vi "Scope Daemon.vi"(0 "Sciscan core Ref":path=path "C:/Users/Laa12/Desktop/SciScan_140404/GFG/GFG_core.ref", 1 "Buttons":T5, 2 "Indicators":T2, 3 "Visualization Parameters":T6, 5 "Current Frame":T1, 7 "Frame Time Stamp":refnum<vi>, 11 "error in (no error)":errorcluster, 12 "Transformation Matrix":refnum<vi>, 13 "FOV controls":T4, 14 "Parameters for Legal Movements":T3) -> (4 "Current Frame Out":T1, 15 "error out":errorcluster)   [LabVIEW 2012, in "Sciscan Scope Daemon.lvlib"]
uses:
  Sciscan Scope Daemon.lvlib
  <vilib>/Analysis/Matrix/Datatypes/RealMatrix.ctl
  <vilib>/vision/Image Controls.llb/IMAQ Image.ctl
  <vilib>/Analysis/Matrix/NI_Matrix.lvlib
panel:
  out "Exit":bool
  out "Image Out":T1
  out "FOVs":dbl[][](array[numeric])
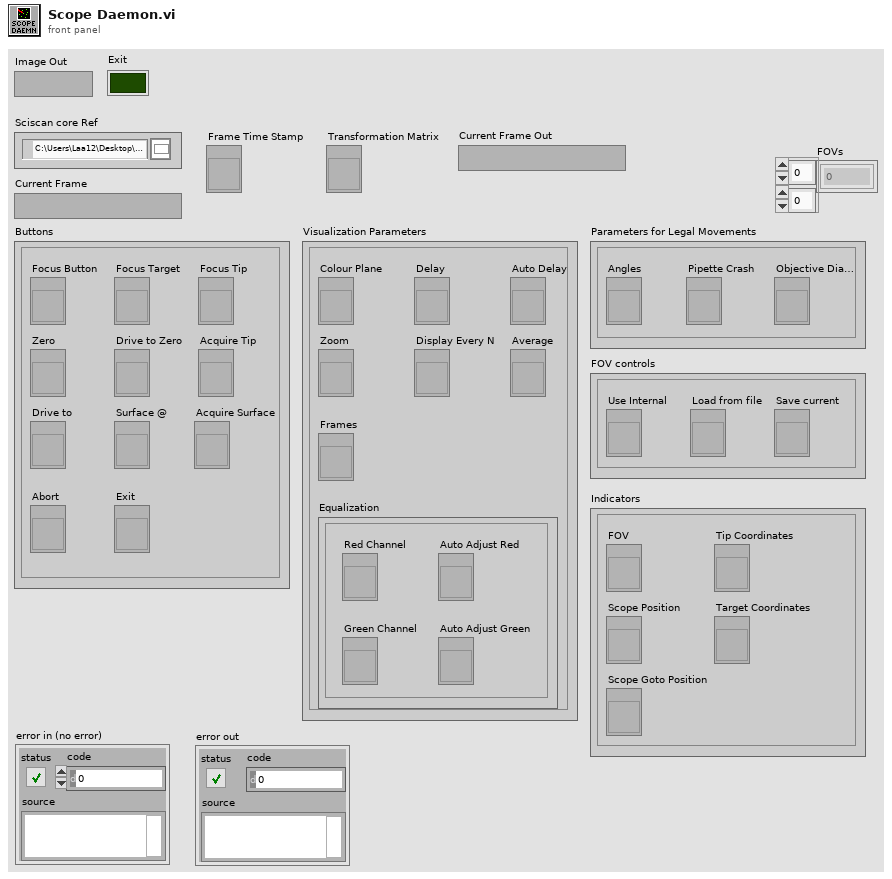
[diagram p1: front panel]
types:
  T1 = typedef "IMAQ Image.ctl" = refnum<image>
  T2 = cluster{"Tip Coordinates":refnum<vi>, "Target Coordinates":refnum<vi>, "Scope Position":refnum<vi>, "FOV":refnum<vi>, "Scope Goto Position":refnum<vi>}
  T3 = cluster{"Angles":refnum<vi>, "Objective Diameter":refnum<vi>, "Pipette Crash":refnum<vi>}
  T4 = cluster{"Use Internal":refnum<vi>, "Load from file":refnum<vi>, "Save current":refnum<vi>}
  T5 = cluster{"Focus Tip":refnum<vi>, "Focus Target":refnum<vi>, "Drive to Zero":refnum<vi>, "Zero":refnum<vi>, "Acquire Tip":refnum<vi>, "Focus Button":refnum<vi>, "Exit":refnum<vi>, "Abort":refnum<vi>, "Drive to":refnum<vi>, "Surface @":refnum<vi>, "Acquire Surface":refnum<vi>}
  T6 = cluster{"Display Every N":refnum<vi>, "Average":refnum<vi>, "Frames":refnum<vi>, "Colour Plane":refnum<vi>, "Zoom":refnum<vi>, "Delay":refnum<vi>, "Equalization":cluster{"Green Channel":refnum<vi>, "Auto Adjust Green":refnum<vi>, "Red Channel":refnum<vi>, "Auto Adjust Red":refnum<vi>}, "Auto Delay":refnum<vi>}
  T7 = cluster{"X [um]":dbl, "Y [um]":dbl, "Z [um]":dbl}
  T8 = typedef "NI_Matrix.lvlib/RealMatrix.ctl" = dbl[][]
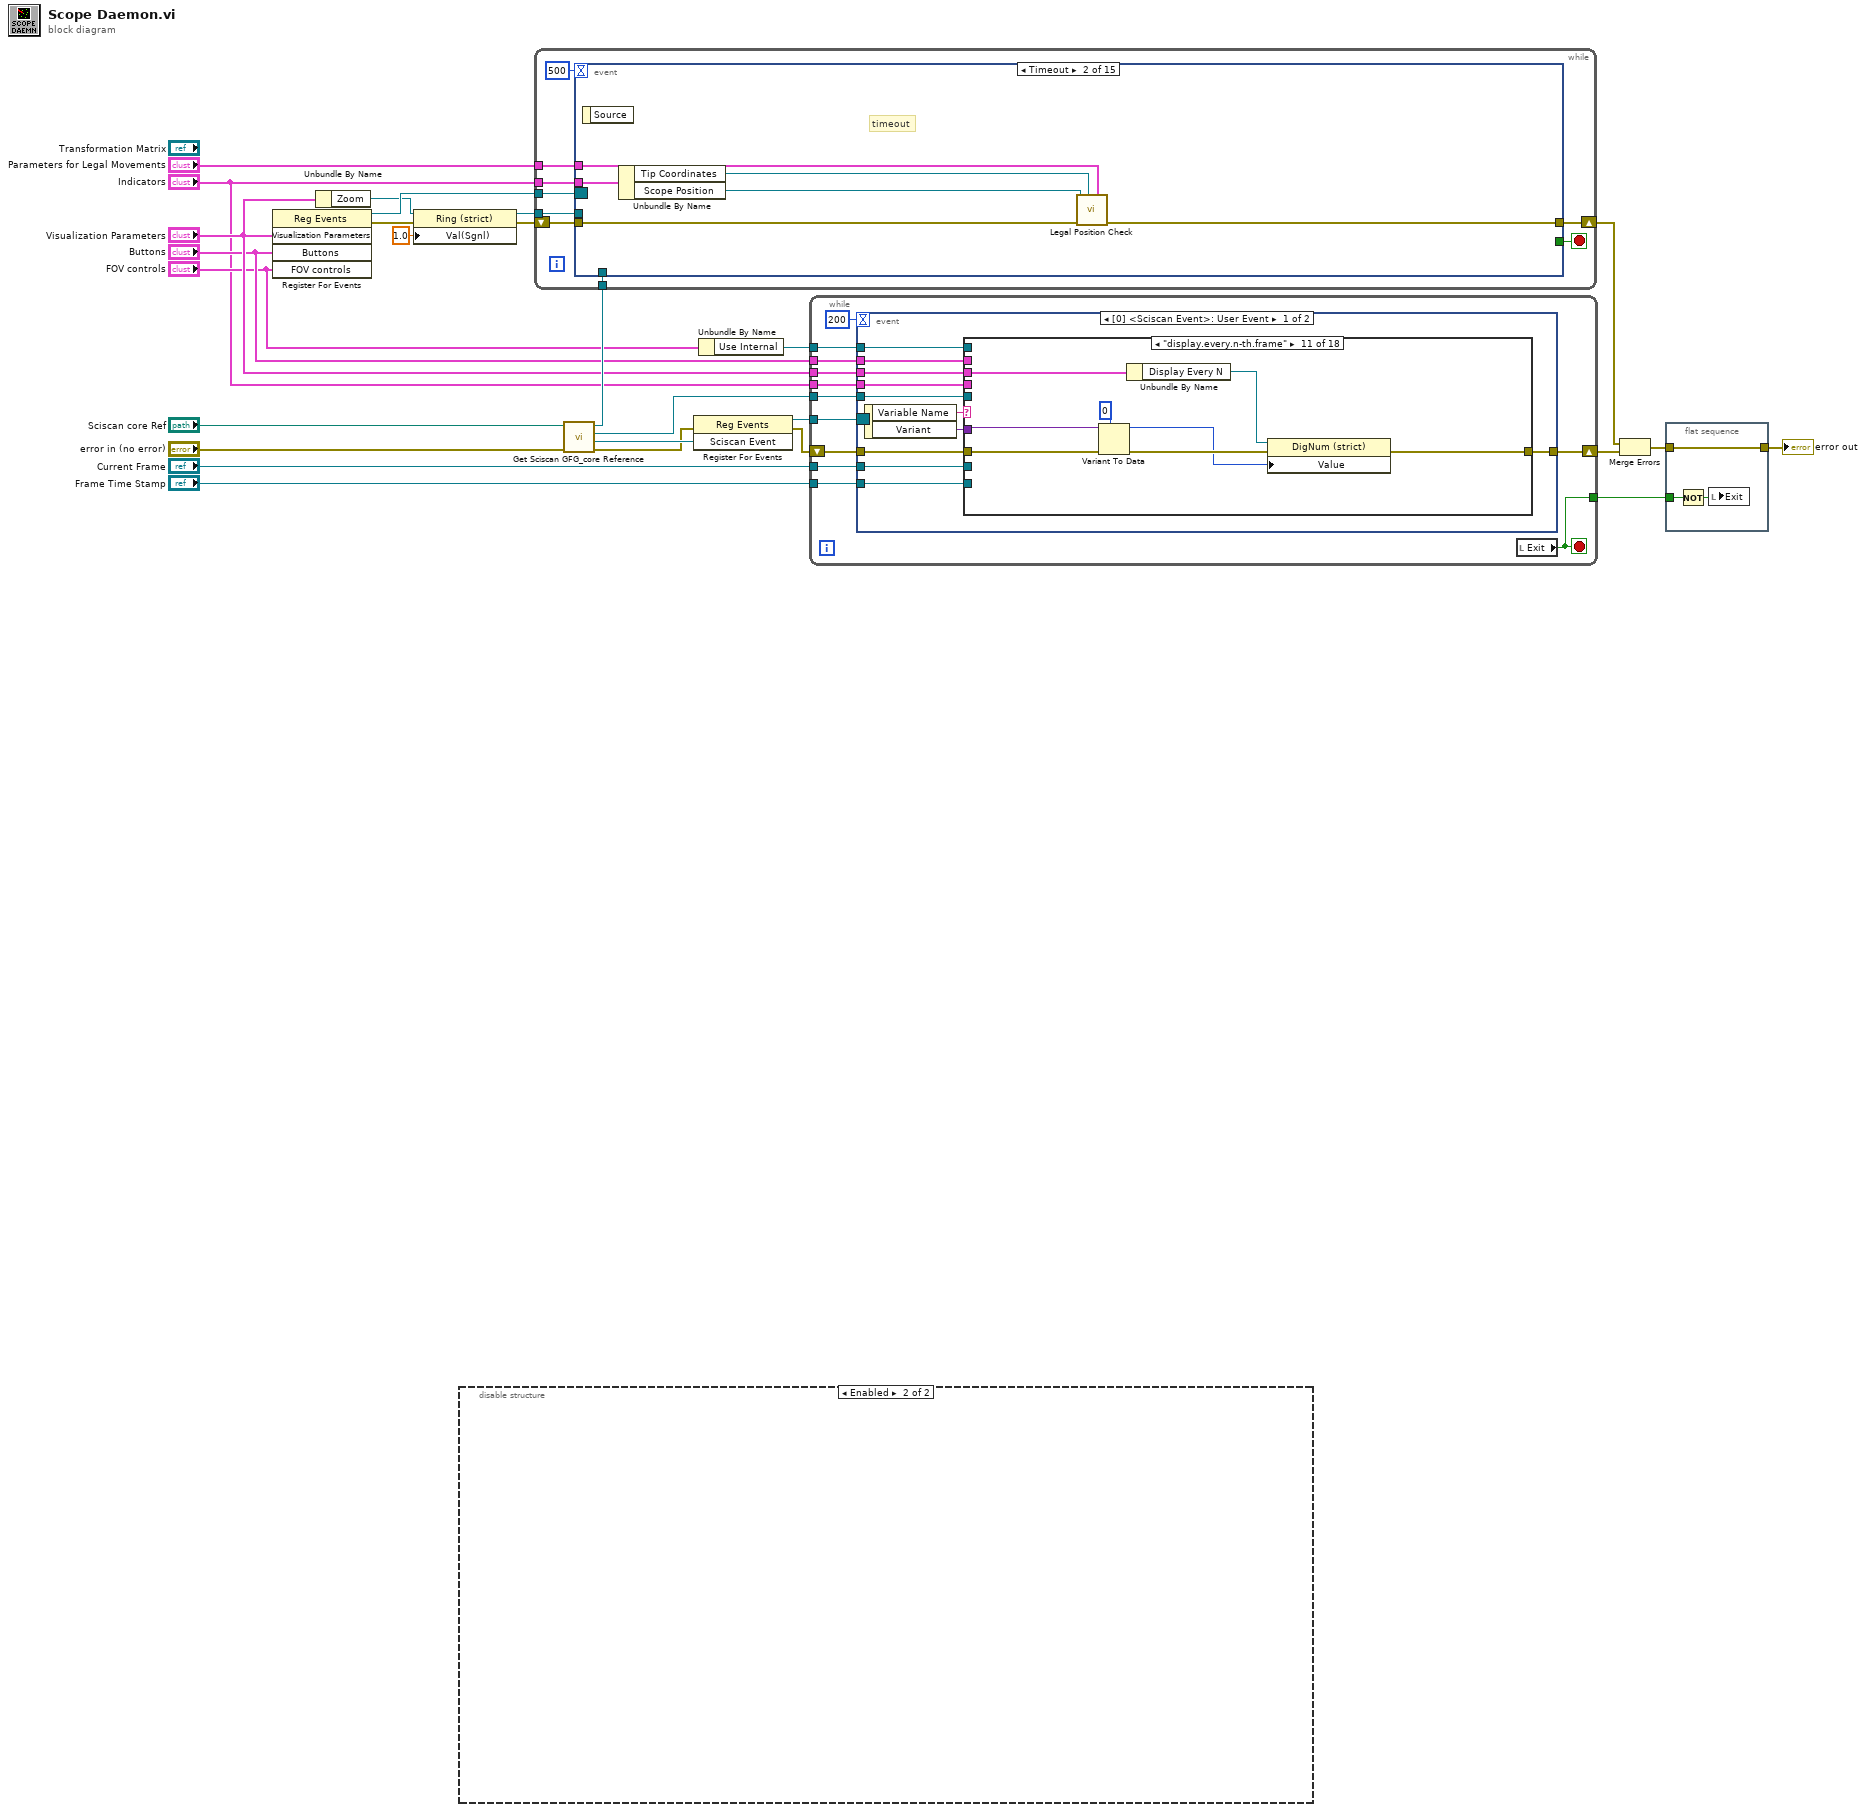
[diagram p0: block diagram]
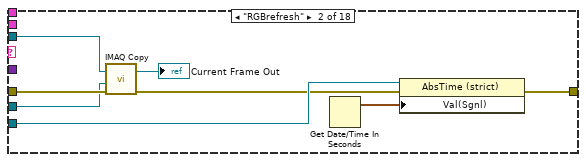
[diagram p3: hidden frame]
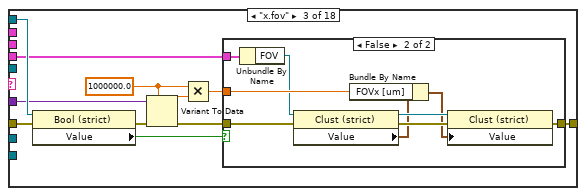
[diagram p4: hidden frame]
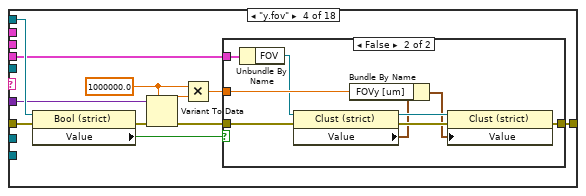
[diagram p6: hidden frame]
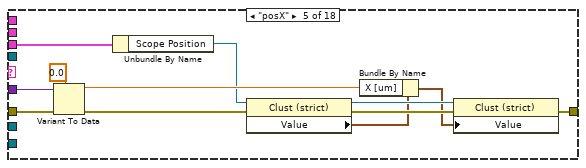
[diagram p8: hidden frame]
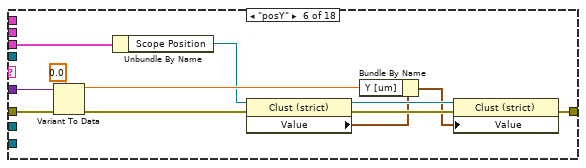
[diagram p9: hidden frame]
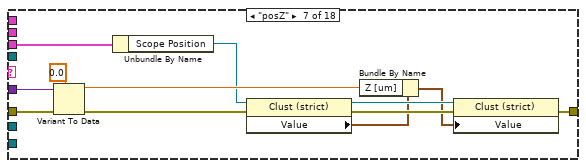
[diagram p10: hidden frame]
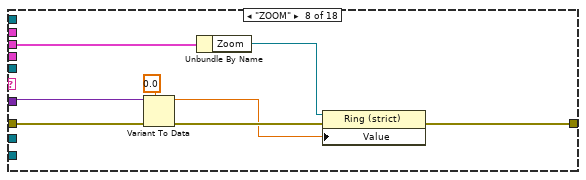
[diagram p11: hidden frame]
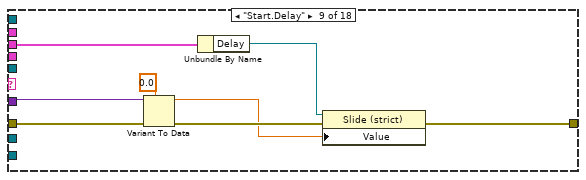
[diagram p12: hidden frame]
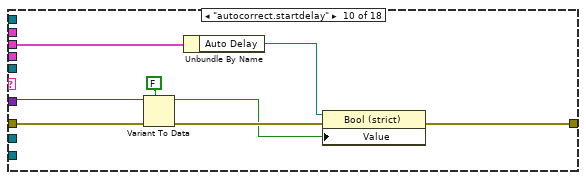
[diagram p13: hidden frame]
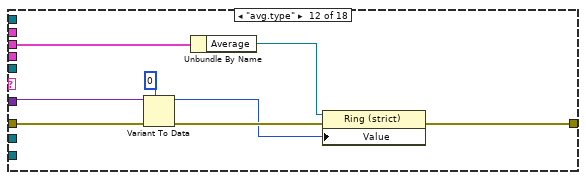
[diagram p14: hidden frame]
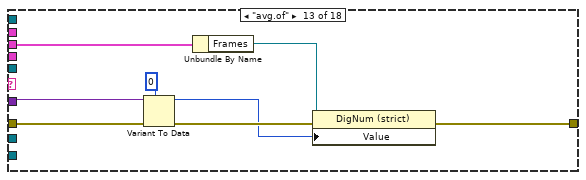
[diagram p15: hidden frame]
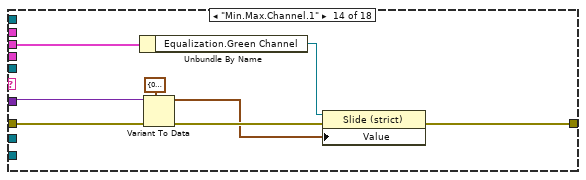
[diagram p16: hidden frame]
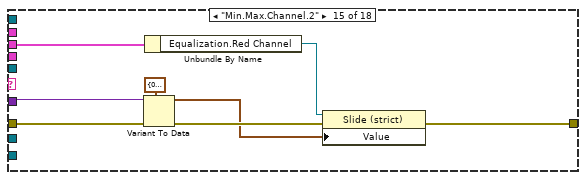
[diagram p17: hidden frame]
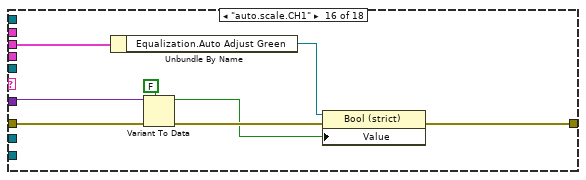
[diagram p18: hidden frame]
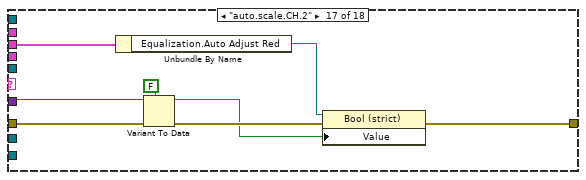
[diagram p19: hidden frame]
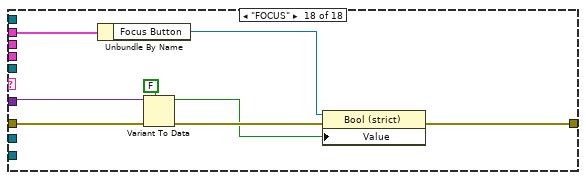
[diagram p20: hidden frame]
diagram:
  n1 = register-events("Visualization Parameters", "Buttons", "FOV controls") -> (reference out=w27:refnum<event-registration>, error out=w24:errorcluster)  [unwired: 2 in]
  n2 = Unbundle By Name("Visualization Parameters") -> ("Zoom"=w23:refnum<vi>)
  n3 = property class="Ring (strict)"(reference=w23, error in=w24, "Val(Sgnl)"=1.0 ("Value (Signaling)")) -> (reference out=w25:refnum<vi>, error out=w19:errorcluster)
  n4 = disable-structure shown="Enabled" {
    frame Disabled {
      n5 = List Folder(path=path "C:/Users/LAA12/Desktop/imagesRGB" ("Images Folder")) -> (path out=w37:path, filenames=w33:string[], error out=w30:errorcluster)  [unwired: 1 in, 3 out]
      n6 = call "IMAQ Create"("Image Name"="Current Image", "error in (no error)"=w30) -> ("New Image"=w40:T1, "error out"=w29:errorcluster)  [unwired: 2 in, 1 out]
      n7 = Delete From Array(array=w33, index=0) -> (array with subset deleted=w35:string[])  [unwired: 1 in, 1 out]
      n8 = Array Size(array=w35) -> (size(s)=w36:i32)
      n9 = Decrement(x=w36) -> (x-1=w32:i32)
      n10 = while {
        tunnel: w40 -> [w55]
        tunnel: w32 -> [w45]
        shift-right: [w50] -> _
        shift-left: u32 0 -> [w47]
        shift-right: [w43] -> w34
        shift-left: w29 -> [w58]
        tunnel: w37 -> [w57]
        tunnel: w35 -> [w56]
        tunnel: [w44] -> w28
        stop <- FALSE stop-if-true
        n11 = Index Array(array=w56, index=w47) -> (element=w54:string)
        n12 = Increment(x=w47) -> (x+1=w46:u32)
        n13 = Build Path(base path=w57, name or relative path=w54) -> (appended path=w53:path)
        n14 = call "IMAQ ReadFile"("File Path"=w53, "error in (no error)"=w58, "Image"=w55) -> ("error out"=w43:errorcluster, "Image Out"=w44:T1)  [unwired: 2 in, 5 out]
        "Image Out" <- w44
        n15 = Less?(x=w46, y=w45) -> (x < y?=w52:bool)
        n16 = Wait (ms)(milliseconds to wait=u32 500) -> ()  [unwired: 1 out]
        n17 = Select(t=w46, s=w52, f=u32 0) -> (s? t:f=w50:u32)
      }
      n18 = call "IMAQ Dispose"("Image"=w28, "error in (no error)"=w34) -> ("error out"=w41:errorcluster)  [unwired: 1 in, 3 out]
      n19 = call <vilib>:"Simple Error Handler.vi"("error in (no error)"=w41) -> ()  [unwired: 1 in, 8 out]
    }
    frame Enabled {
    }
  }
  n20 = call "Get Sciscan GFG_core Reference.vi"("error in"="error in (no error)", "file path"="Sciscan core Ref") -> ("error out"=w10:errorcluster, "Sciscan Event"=w11:refnum<user-event>, "RGB overlay"=w14:T1, "GFG reference"=w17:refnum<vi>)  [unwired: 6 in]
  n21 = while {
    tunnel: w27 -> [w67]
    shift-right: [w66] -> w4
    shift-left: w19 -> [w65]
    tunnel: w25 -> [w63]
    tunnel: w17 -> [w59]
    tunnel: "Parameters for Legal Movements" -> [w61]
    tunnel: "Indicators" -> [w60]
    stop <- w64 stop-if-true
    n22 = event shown="[1] Timeout" {
      selector: w67 -> [_ _ _ _ _ _ _ _ _ _ _ _ _ _ _]
      dyn-events: _ -> [_ _ _ _ _ _ _ _ _ _ _ _ _ _ _]
      timeout: 500 -> [_ _ _ _ _ _ _ _ _ _ _ _ _ _ _]
      tunnel: [w74 w94 w108 w117 w137 w143 w198 w214 w231 w242 w246 w250 w252 w267 w271] -> w66
      tunnel: w65 -> [w71 w99 w103 w116 w134 w146 w199 w213 w239 w243 w245 w251 w255 w259 w271]
      tunnel: [_ _ _ _ _ _ _ _ _ _ _ _ _ _ TRUE] -> w64
      tunnel: w63 -> [_ _ _ _ _ w144 _ _ _ _ _ _ _ _ _]
      tunnel: w61 -> [_ w98 _ _ _ _ _ _ _ _ _ _ _ _ _]
      tunnel: w60 -> [_ w97 _ _ _ _ _ _ _ _ _ _ _ w262 _]
      tunnel: w59 -> [w73 _ w104 w115 w135 w145 _ w212 w229 w241 w247 w249 w254 _ _]
      event Value Change {
        # "dynamics"
        # "focus target\nfocus tip"
        n23 = event-data() -> ("CtlRef"=w75:refnum<vi>)  [unwired: 1 in]
        n24 = local read "Visualization Parameters"() -> (w70:T6)
        n25 = local read "Buttons"() -> (w77:T5)
        n26 = local read "Indicators"() -> (w79:T2)
        n27 = Unbundle By Name(w70) -> ("Zoom"=w69:refnum<vi>)
        n28 = Unbundle By Name(w77) -> ("Focus Target"=w78:refnum<vi>)
        n29 = Unbundle By Name(w79) -> ("Target Coordinates"=w82:refnum<vi>, "Tip Coordinates"=w83:refnum<vi>, "FOV"=w84:refnum<vi>)
        n30 = property class="Ring (strict)"(reference=w69, error in=w71) -> (error out=w72:errorcluster, "Value"=w68:dbl)  [unwired: 1 out]
        n31 = local read "Transformation Matrix"() -> (w76:refnum<vi>)
        n32 = property class="Clust (strict)"(reference=w84) -> (error out=w93:errorcluster, "Value"=w86:cluster{"FOVx [um]":dbl, "FOVy [um]":dbl})  [unwired: 1 in, 1 out]
        n33 = Equal?(x=w78, y=w75) -> (x = y?=w92:bool)
        n34 = Select(t=w82, s=w92, f=w83) -> (s? t:f=w90:refnum<vi>)
        n35 = property class="Clust (strict)"(reference=w90, error in=w93) -> (error out=w89:errorcluster, "Value"=w85:T7)  [unwired: 1 out]
        n36 = property class="Arr (strict)"(reference=w76, error in=w72) -> (error out=w81:errorcluster, "Value"=w80:T8)  [unwired: 1 out]
        n37 = call "Focus Point.vi"("Zoom Factor"=w68, "Transformation Matrix"=w80, "error in"=w81, "FOV"=w86, "Target Coordinates"=w85, "GFG Refnum"=w73) -> ("error out"=w91:errorcluster)  [unwired: 4 in, 1 out]
        n38 = property class="Bool (strict)"(reference=w75, error in=w89, "Value"=FALSE) -> (error out=w87:errorcluster)  [unwired: 1 out]
        n39 = Merge Errors(w87, w91) -> (w74:errorcluster)
      }
      event Timeout {
        # "timeout"
        n40 = event-data() -> ()  [unwired: 1 in, 1 out]
        n41 = Unbundle By Name(w97) -> ("Tip Coordinates"=w96:refnum<vi>, "Scope Position"=w95:refnum<vi>)
        n42 = call "Legal Position Check.vi"("Parameters for Legal Movements"=w98, "error in (no error)"=w99, "Scope Position"=w95, "Tip Coordinates"=w96) -> ("error out"=w94:errorcluster)  [unwired: 6 in, 1 out]
      }
      event Value Change {
        # "drive to position"
        n43 = event-data() -> ()  [unwired: 1 in, 3 out]
        n44 = call "Set Sciscan Dynamics.vi"("error in"=w103, "Fast"=FALSE, "GFG Refnum"=w104) -> ("error out"=w102:errorcluster, "GFG Refnum Out"=w101:refnum<vi>)  [unwired: 7 in]
        n45 = local read "Buttons"() -> (w107:T5)
        n46 = local read "Indicators"() -> (w113:T2)
        n47 = Unbundle By Name(w107) -> ("Drive to"=w106:refnum<vi>)
        n48 = Unbundle By Name(w113) -> ("Scope Goto Position"=w112:refnum<vi>)
        n49 = property on="Property Node" class="Clust (strict)"(reference=w112, error in=w102) -> (error out=w111:errorcluster, "Value"=w110:T7)  [unwired: 1 out]
        n50 = call "Move Sciscan Scope.vi"("Type"=enum16{"Relative", "Absolute"}."Absolute", "error in"=w111, "Displacement [um]"=w110, "GFG Refnum"=w101) -> ("error out"=w109:errorcluster)  [unwired: 6 in, 1 out]
        n51 = property on="Property Node" class="Bool (strict)"(reference=w106, error in=w109, "Value"=FALSE) -> (error out=w108:errorcluster)  [unwired: 1 out]
      }
      event Value Change {
        # "zero"
        n52 = event-data() -> ("CtlRef"=w118:refnum<vi>)  [unwired: 1 in]
        n53 = flat-sequence {
          tunnel: w116 -> [w125]
          tunnel: w115 -> [w126]
          tunnel: [w126] -> w123
          tunnel: [w125] -> w122
          tunnel: [w127] -> w121
          tunnel: w123 -> [w129]
          tunnel: w122 -> [w128]
          tunnel: [w131] -> w120
          tunnel: w121 -> [w131]
          frame #0 {
            n54 = Wait (ms)(milliseconds to wait=u32 1000) -> ()  [unwired: 1 out]
          }
          frame #1 {
            n55 = call "Zero.vi"("error in"=w128, "GFG Refnum"=w129) -> ("error out"=w127:errorcluster)  [unwired: 8 in, 1 out]
          }
          frame #2 {
            n56 = Wait (ms)(milliseconds to wait=u32 2000) -> ()  [unwired: 1 out]
          }
        }
        n57 = property on="Property Node" class="Bool (strict)"(reference=w118, error in=w120, "Value"=FALSE) -> (error out=w117:errorcluster)  [unwired: 1 out]
      }
      event Value Change {
        # "dynamics"
        # "drive to zero"
        n58 = event-data() -> ("CtlRef"=w138:refnum<vi>)  [unwired: 1 in]
        n59 = call "Set Sciscan Dynamics.vi"("error in"=w134, "Fast"=FALSE, "GFG Refnum"=w135) -> ("error out"=w133:errorcluster, "GFG Refnum Out"=w132:refnum<vi>)  [unwired: 7 in]
        n60 = call "Move Sciscan Scope.vi"("Type"=enum16{"Relative", "Absolute"}."Absolute", "error in"=w133, "Displacement [um]"=T7 {"X [um]"=0.0, "Y [um]"=0.0, "Z [um]"=0.0}, "GFG Refnum"=w132) -> ("error out"=w140:errorcluster)  [unwired: 6 in, 1 out]
        n61 = property on="Property Node" class="Bool (strict)"(reference=w138, error in=w140, "Value"=FALSE) -> (error out=w137:errorcluster)  [unwired: 1 out]
      }
      event Value Change {
        # "zoom\nuse internal"
        n62 = event-data() -> ()  [unwired: 1 in, 1 out]
        n63 = local read "FOV controls"() -> (w151:T4)
        n64 = Unbundle By Name(w151) -> ("Use Internal"=w150:refnum<vi>)
        n65 = property class="Ring (strict)"(reference=w144, error in=w146) -> (reference out=w152:refnum<vi>, error out=w160:errorcluster, "Value"=w159:dbl)
        n66 = property class="Bool (strict)"(reference=w150) -> (error out=w147:errorcluster, "Value"=w153:bool)  [unwired: 1 in, 1 out]
        n67 = call "Set Sciscan Scope Zoom.vi"("error in"=w160, "Zoom"=w159, "GFG Refnum"=w145) -> ("error out"=w156:errorcluster, "GFG Refnum Out"=w155:refnum<vi>)  [unwired: 7 in]
        n68 = case shown="False" w153 {
          tunnel: w155 -> [w166 _]
          tunnel: [w165 w175] -> w149
          tunnel: w156 -> [w164 w178]
          tunnel: [w161 w186] -> w158
          tunnel: w152 -> [_ w185]
          frame False {
            n69 = flat-sequence {
              tunnel: w164 -> [w168]
              tunnel: w166 -> [w169]
              tunnel: [w169] -> w163
              tunnel: [w168] -> w162
              tunnel: [w172] -> w165
              tunnel: [w170] -> w161
              tunnel: w163 -> [w173]
              tunnel: w162 -> [w171]
              frame #0 {
                n70 = Wait (ms)(milliseconds to wait=u32 2000) -> ()  [unwired: 1 out]
              }
              frame #1 {
                n71 = call "Get Sciscan FOV.vi"("error in"=w171, "GFG Refnum"=w173) -> ("error out"=w172:errorcluster, "FOV"=w170:cluster{"Width [um]":dbl, "Height [um]":dbl})  [unwired: 7 in, 1 out]
              }
            }
          }
          frame True {
            w183 = 0 ("index (row)")
            n72 = local read "FOVs"() -> (w174:dbl[][])
            n73 = Index Array(array=w174, index (row)=w183, index (col)=w183) -> (element=w182:dbl)
            n74 = Not A Number/Path/Refnum?(number/path/refnum=w182) -> (NaN/Path/Refnum?=w181:bool)
            n75 = Less Or Equal To 0?(x=w182) -> (x <= 0?=w180:bool)
            n76 = Or(x=w181, y=w180) -> (x .or. y?=w179:bool)
            n77 = case shown="True" w179 {
              tunnel: [w193 w196] -> w177
              tunnel: w178 -> [w193 w195]
              tunnel: [w192 w194] -> w176
              tunnel: w174 -> [w192 _]
              frame False {
              }
              frame True {
                n78 = call "Load Zoom FOV table.vi"("error in"=w195, "Max Zoom"=8) -> ("error out"=w196:errorcluster, "FOVs"=w194:dbl[][])  [unwired: 8 in]
              }
            }
            "FOVs" <- w176
            n79 = property on="Property Node" class="Ring (strict)"(reference=w185, error in=w177) -> (error out=w175:errorcluster, "Value"=w191:dbl)  [unwired: 1 out]
            n80 = Decrement(x=w191) -> (x-1=w184:dbl)
            n81 = Index Array(array=w176, index (row) #1=w184, index (col) #1=1 ("disabled index (col)"), index (row) #2=w184, index (col) #2=2 ("disabled index (col)")) -> (element #1=w188:dbl, element #2=w187:dbl)
            n82 = Bundle("input 3"=w188, "input 3"=w187) -> (w186:cluster{"input 3":dbl, "input 3":dbl})  [unwired: 1 in]
          }
        }
        n83 = local read "Indicators"() -> (w154:T2)
        n84 = Unbundle By Name(w154) -> ("FOV"=w157:refnum<vi>)
        n85 = property on="Property Node" class="Clust (strict)"(reference=w157, error in=w149, "Value"=w158) -> (error out=w148:errorcluster)  [unwired: 1 out]
        n86 = Merge Errors(w147, w148) -> (w143:errorcluster)
      }
      event Value Change {
        # "load from file"
        n87 = event-data() -> ("CtlRef"=w200:refnum<vi>)  [unwired: 1 in]
        n88 = local read "Visualization Parameters"() -> (w201:T6)
        n89 = local read "Indicators"() -> (w210:T2)
        n90 = Unbundle By Name(w201) -> ("Zoom"=w207:refnum<vi>)
        n91 = Unbundle By Name(w210) -> ("FOV"=w209:refnum<vi>)
        n92 = property class="Clust (strict)"(reference=w209, error in=w199) -> (error out=w208:errorcluster, "Value"=w204:cluster{"FOVx [um]":dbl, "FOVy [um]":dbl})  [unwired: 1 out]
        n93 = property class="Ring (strict)"(reference=w207, error in=w208) -> (error out=w205:errorcluster, "Value"=w206:dbl)  [unwired: 1 out]
        n94 = call "Save Current Fov.vi"("Max Zoom"=8, "error in"=w205, "Current FOV"=w204, "Current Zoom"=w206) -> ("error out"=w203:errorcluster)  [unwired: 6 in, 1 out]
        n95 = property class="Bool (strict)"(reference=w200, error in=w203, "Value"=FALSE) -> (error out=w198:errorcluster)  [unwired: 1 out]
      }
      event Value Change {
        n96 = event-data() -> ()  [unwired: 1 in, 1 out]
        n97 = local read "Visualization Parameters"() -> (w228:T6)
        n98 = Unbundle By Name(w228) -> ("Equalization.Red Channel"=w225:refnum<vi>, "Equalization.Green Channel"=w226:refnum<vi>, "Equalization.Auto Adjust Green"=w221:refnum<vi>, "Equalization.Auto Adjust Red"=w220:refnum<vi>)
        n99 = property class="Slide (strict)"(reference=w226) -> (error out=w227:errorcluster, "Value"=w223:cluster{dbl, dbl})  [unwired: 1 in, 1 out]
        n100 = property class="Bool (strict)"(reference=w220) -> (error out=w222:errorcluster, "Value"=w218:bool)  [unwired: 1 in, 1 out]
        n101 = property class="Slide (strict)"(reference=w225, error in=w227) -> (error out=w216:errorcluster, "Value"=w224:cluster{dbl, dbl})  [unwired: 1 out]
        n102 = property class="Bool (strict)"(reference=w221, error in=w222) -> (error out=w217:errorcluster, "Value"=w219:bool)  [unwired: 1 out]
        n103 = call "Set Sciscan Scope Image Equalization.vi"("Red Channel"=w224, "Green Channel"=w223, "error in"=w213, "Auto Adjust Red"=w218, "Auto Adjust Green"=w219, "GFG Refnum"=w212) -> ("error out"=w215:errorcluster)  [unwired: 4 in, 1 out]
        n104 = Merge Errors(w216, w217, w215) -> (w214:errorcluster)
      }
      event Value Change {
        # "avg\nframes"
        n105 = event-data() -> ()  [unwired: 1 in, 1 out]
        n106 = local read "Visualization Parameters"() -> (w238:T6)
        n107 = Unbundle By Name(w238) -> ("Average"=w237:refnum<vi>, "Frames"=w236:refnum<vi>)
        n108 = property class="DigNum (strict)"(reference=w236) -> (error out=w235:errorcluster, "Value"=w233:i8)  [unwired: 1 in, 1 out]
        n109 = property class="Ring (strict)"(reference=w237, error in=w235) -> (error out=w230:errorcluster, "Value"=w234:u16)  [unwired: 1 out]
        n110 = call "Set Sciscan Scope Image Averaging.vi"("error in"=w239, "Frames"=w233, "Average"=w234, "GFG Refnum"=w229) -> ("error out"=w232:errorcluster)  [unwired: 6 in, 1 out]
        n111 = Merge Errors(w230, w232) -> (w231:errorcluster)
      }
      event Value Change {
        # "display every N"
        n112 = event-data() -> ("NewVal"=w240:i8)  [unwired: 1 in]
        n113 = call "Set Sciscan Scope Image Refresh.vi"("error in"=w243, "display every n-th frame"=w240, "GFG Refnum"=w241) -> ("error out"=w242:errorcluster)  [unwired: 7 in, 1 out]
      }
      event Value Change {
        # "Delay"
        n114 = event-data() -> ("NewVal"=w244:dbl)  [unwired: 1 in]
        n115 = call "Set Sciscan Scope Image Delay.vi"("error in"=w245, "Delay"=w244, "GFG Refnum"=w247) -> ("error out"=w246:errorcluster)  [unwired: 7 in, 1 out]
      }
      event Value Change {
        # "Delay"
        n116 = event-data() -> ("NewVal"=w248:bool)  [unwired: 1 in]
        n117 = call "Auto Sciscan Scope Image Delay.vi"("error in"=w251, "Auto Delay"=w248, "GFG Refnum"=w249) -> ("error out"=w250:errorcluster)  [unwired: 7 in, 1 out]
      }
      event Value Change {
        # "focus"
        n118 = event-data() -> ("NewVal"=w253:bool)  [unwired: 1 in]
        n119 = call "Set Sciscan Scope Focus.vi"("error in"=w255, "Focus Button"=w253, "GFG Refnum"=w254) -> ("error out"=w252:errorcluster)  [unwired: 7 in, 1 out]
      }
      event "Buttons.Acquire Surface": Value Change {
        n120 = event-data() -> ()  [unwired: 1 in, 1 out]
        n121 = local read "Buttons"() -> (w266:T5)
        n122 = Unbundle By Name(w266) -> ("Acquire Surface"=w265:refnum<vi>, "Surface @"=w261:refnum<vi>)
        n123 = Unbundle By Name(w262) -> ("Scope Position"=w258:refnum<vi>)
        n124 = property on="Property Node" class="Clust (strict)"(reference=w258, error in=w259) -> (error out=w260:errorcluster, "Value"=w257:T7)  [unwired: 1 out]
        n125 = Unbundle By Name(w257) -> ("Z [um]"=w256:dbl)
        n126 = property on="Property Node" class="DigNum (strict)"(reference=w261, error in=w260, "Value"=w256) -> (error out=w263:errorcluster)  [unwired: 1 out]
        n127 = property on="Property Node" class="Bool (strict)"(reference=w265, error in=w263, "Value"=FALSE) -> (error out=w267:errorcluster)  [unwired: 1 out]
      }
      event Value Change {
        # "exit"
        n128 = event-data() -> ()  [unwired: 1 in, 1 out]
        n129 = local write "FOVs"(dbl[][] [] ("Array")) -> ()
        "Exit" <- TRUE ("Exit")
      }
    }
  }
  n130 = register-events(error in=w10, w11) -> (reference out=w18:refnum<event-registration>, error out=w12:errorcluster)  [unwired: 1 in]
  n131 = Unbundle By Name("FOV controls") -> ("Use Internal"=w16:refnum<vi>)
  n132 = while {
    tunnel: w18 -> [w283]
    tunnel: w16 -> [w282]
    shift-right: [w280] -> w5
    shift-left: w12 -> [w281]
    tunnel: "Indicators" -> [w279]
    tunnel: "Visualization Parameters" -> [w278]
    tunnel: "Frame Time Stamp" -> [w277]
    tunnel: w14 -> [w276]
    tunnel: "Current Frame" -> [w275]
    tunnel: "Buttons" -> [w274]
    tunnel: [w273] -> w1
    stop <- w273 stop-if-true
    n133 = event shown="[0] <Sciscan Event>: User Event" {
      selector: w283 -> [_ _]
      dyn-events: _ -> [_ _]
      timeout: 200 -> [_ _]
      tunnel: w282 -> [w293 _]
      tunnel: w281 -> [w292 w470]
      tunnel: [w291 w470] -> w280
      tunnel: w279 -> [w290 _]
      tunnel: w278 -> [w289 _]
      tunnel: w277 -> [w287 _]
      tunnel: w276 -> [w286 _]
      tunnel: w275 -> [w285 _]
      tunnel: w274 -> [w284 _]
      event User Event {
        n134 = event-data() -> ("Variable Name"=w288:string, "Variant"=w294:variant)  [unwired: 1 in]
        n135 = case shown="\"display.every.n-th.frame\"" w288 {
          tunnel: w294 -> [_ _ w311 w332 w357 w369 w381 w388 w396 w404 w412 w420 w428 w436 w444 w452 w460 w468]
          tunnel: w293 -> [_ _ w313 w334 _ _ _ _ _ _ _ _ _ _ _ _ _ _]
          tunnel: w292 -> [w295 w301 w312 w333 w346 w358 w370 w389 w397 w405 w413 w421 w429 w437 w445 w453 w461 w469]
          tunnel: [w295 w302 w306 w327 w355 w367 w379 w386 w394 w402 w410 w418 w426 w434 w442 w450 w458 w466] -> w291
          tunnel: w290 -> [_ _ w304 w325 w354 w366 w378 _ _ _ _ _ _ _ _ _ _ _]
          tunnel: w289 -> [_ _ _ _ _ _ _ w385 w393 w401 w409 w417 w425 w433 w441 w449 w457 _]
          tunnel: w287 -> [_ w303 _ _ _ _ _ _ _ _ _ _ _ _ _ _ _ _]
          tunnel: w286 -> [_ w300 _ _ _ _ _ _ _ _ _ _ _ _ _ _ _ _]
          tunnel: w285 -> [_ w299 _ _ _ _ _ _ _ _ _ _ _ _ _ _ _ _]
          tunnel: w284 -> [_ _ _ _ _ _ _ _ _ _ _ _ _ _ _ _ _ w462]
          frame "False", Default {
          }
          frame "RGBrefresh" {
            n136 = call "IMAQ Copy"("error in (no error)"=w301, "Image Dst"=w299, "Image Src"=w300) -> ("error out"=w297:errorcluster, "Image Dst Out"=→"Current Frame Out":T1)  [unwired: 3 out]
            n137 = Get Date/Time In Seconds() -> (seconds since 1Jan1904=w298:timestamp)
            n138 = property on="Property Node" class="AbsTime (strict)"(reference=w303, error in=w297, "Val(Sgnl)"=w298) -> (error out=w302:errorcluster)  [unwired: 1 out]
          }
          frame "x.fov" {
            w308 = 1000000.0
            n139 = property class="Bool (strict)"(reference=w313, error in=w312) -> (error out=w310:errorcluster, "Value"=w314:bool)  [unwired: 1 out]
            n140 = Variant To Data(error in=w310, type=w308, Variant=w311) -> (data=w305:dbl, error out=w309:errorcluster)
            n141 = Multiply(x=w308, y=w305) -> (x*y=w307:dbl)
            n142 = case shown="False" w314 {
              tunnel: [w315 w324] -> w306
              tunnel: w309 -> [w315 w323]
              tunnel: w307 -> [_ w320]
              tunnel: w304 -> [_ w316]
              frame True {
              }
              frame False {
                n143 = Unbundle By Name(w316) -> ("FOV"=w317:refnum<vi>)
                n144 = property on="Property Node" class="Clust (strict)"(reference=w317, error in=w323) -> (reference out=w321:refnum<vi>, error out=w322:errorcluster, "Value"=w319:cluster{"FOVx [um]":dbl, "FOVy [um]":dbl})
                n145 = Bundle By Name(cluster=w319, "FOVx [um]"=w320) -> (w318:cluster{"FOVx [um]":dbl, "FOVy [um]":dbl})
                n146 = property on="Property Node" class="Clust (strict)"(reference=w321, error in=w322, "Value"=w318) -> (error out=w324:errorcluster)  [unwired: 1 out]
              }
            }
          }
          frame "y.fov" {
            w329 = 1000000.0
            n147 = property class="Bool (strict)"(reference=w334, error in=w333) -> (error out=w331:errorcluster, "Value"=w335:bool)  [unwired: 1 out]
            n148 = Variant To Data(error in=w331, type=w329, Variant=w332) -> (data=w326:dbl, error out=w330:errorcluster)
            n149 = Multiply(x=w329, y=w326) -> (x*y=w328:dbl)
            n150 = case shown="False" w335 {
              tunnel: [w336 w345] -> w327
              tunnel: w330 -> [w336 w344]
              tunnel: w328 -> [_ w341]
              tunnel: w325 -> [_ w337]
              frame True {
              }
              frame False {
                n151 = Unbundle By Name(w337) -> ("FOV"=w338:refnum<vi>)
                n152 = property on="Property Node" class="Clust (strict)"(reference=w338, error in=w344) -> (reference out=w342:refnum<vi>, error out=w343:errorcluster, "Value"=w340:cluster{"FOVx [um]":dbl, "FOVy [um]":dbl})
                n153 = Bundle By Name(cluster=w340, "FOVy [um]"=w341) -> (w339:cluster{"FOVx [um]":dbl, "FOVy [um]":dbl})
                n154 = property on="Property Node" class="Clust (strict)"(reference=w342, error in=w343, "Value"=w339) -> (error out=w345:errorcluster)  [unwired: 1 out]
              }
            }
          }
          frame "posX" {
            n155 = Variant To Data(error in=w346, type=0.0 ("X [um]"), Variant=w357) -> (data=w352:dbl, error out=w356:errorcluster)
            n156 = Unbundle By Name(w354) -> ("Scope Position"=w347:refnum<vi>)
            n157 = property on="Property Node" class="Clust (strict)"(reference=w347, error in=w356) -> (reference out=w350:refnum<vi>, error out=w351:errorcluster, "Value"=w349:T7)
            n158 = Bundle By Name(cluster=w349, "X [um]"=w352) -> (w348:T7)
            n159 = property on="Property Node" class="Clust (strict)"(reference=w350, error in=w351, "Value"=w348) -> (error out=w355:errorcluster)  [unwired: 1 out]
          }
          frame "posY" {
            n160 = Variant To Data(error in=w358, type=0.0 ("X [um]"), Variant=w369) -> (data=w364:dbl, error out=w368:errorcluster)
            n161 = Unbundle By Name(w366) -> ("Scope Position"=w359:refnum<vi>)
            n162 = property on="Property Node" class="Clust (strict)"(reference=w359, error in=w368) -> (reference out=w362:refnum<vi>, error out=w363:errorcluster, "Value"=w361:T7)
            n163 = Bundle By Name(cluster=w361, "Y [um]"=w364) -> (w360:T7)
            n164 = property on="Property Node" class="Clust (strict)"(reference=w362, error in=w363, "Value"=w360) -> (error out=w367:errorcluster)  [unwired: 1 out]
          }
          frame "posZ" {
            n165 = Variant To Data(error in=w370, type=0.0 ("X [um]"), Variant=w381) -> (data=w376:dbl, error out=w380:errorcluster)
            n166 = Unbundle By Name(w378) -> ("Scope Position"=w371:refnum<vi>)
            n167 = property on="Property Node" class="Clust (strict)"(reference=w371, error in=w380) -> (reference out=w374:refnum<vi>, error out=w375:errorcluster, "Value"=w373:T7)
            n168 = Bundle By Name(cluster=w373, "Z [um]"=w376) -> (w372:T7)
            n169 = property on="Property Node" class="Clust (strict)"(reference=w374, error in=w375, "Value"=w372) -> (error out=w379:errorcluster)  [unwired: 1 out]
          }
          frame "ZOOM" {
            n170 = Variant To Data(error in=w389, type=0.0 ("display every n-th frame"), Variant=w388) -> (data=w383:dbl, error out=w387:errorcluster)
            n171 = Unbundle By Name(w385) -> ("Zoom"=w384:refnum<vi>)
            n172 = property on="Property Node" class="Ring (strict)"(reference=w384, error in=w387, "Value"=w383) -> (error out=w386:errorcluster)  [unwired: 1 out]
          }
          frame "Start.Delay" {
            n173 = Variant To Data(error in=w397, type=0.0 ("display every n-th frame"), Variant=w396) -> (data=w391:dbl, error out=w395:errorcluster)
            n174 = Unbundle By Name(w393) -> ("Delay"=w392:refnum<vi>)
            n175 = property on="Property Node" class="Slide (strict)"(reference=w392, error in=w395, "Value"=w391) -> (error out=w394:errorcluster)  [unwired: 1 out]
          }
          frame "autocorrect.startdelay" {
            n176 = Variant To Data(error in=w405, type=FALSE, Variant=w404) -> (data=w399:bool, error out=w403:errorcluster)
            n177 = Unbundle By Name(w401) -> ("Auto Delay"=w400:refnum<vi>)
            n178 = property on="Property Node" class="Bool (strict)"(reference=w400, error in=w403, "Value"=w399) -> (error out=w402:errorcluster)  [unwired: 1 out]
          }
          frame "display.every.n-th.frame" {
            n179 = Variant To Data(error in=w413, type=i8 0 ("Value"), Variant=w412) -> (data=w406:i8, error out=w411:errorcluster)
            n180 = Unbundle By Name(w409) -> ("Display Every N"=w408:refnum<vi>)
            n181 = property on="Property Node" class="DigNum (strict)"(reference=w408, error in=w411, "Value"=w406) -> (error out=w410:errorcluster)  [unwired: 1 out]
          }
          frame "avg.type" {
            n182 = Variant To Data(error in=w421, type=u16 0 ("Value"), Variant=w420) -> (data=w414:u16, error out=w419:errorcluster)
            n183 = Unbundle By Name(w417) -> ("Average"=w416:refnum<vi>)
            n184 = property on="Property Node" class="Ring (strict)"(reference=w416, error in=w419, "Value"=w414) -> (error out=w418:errorcluster)  [unwired: 1 out]
          }
          frame "avg.of" {
            n185 = Variant To Data(error in=w429, type=i8 0 ("Value"), Variant=w428) -> (data=w422:i8, error out=w427:errorcluster)
            n186 = Unbundle By Name(w425) -> ("Frames"=w424:refnum<vi>)
            n187 = property on="Property Node" class="DigNum (strict)"(reference=w424, error in=w427, "Value"=w422) -> (error out=w426:errorcluster)  [unwired: 1 out]
          }
          frame "Min.Max.Channel.1" {
            n188 = Unbundle By Name(w433) -> ("Equalization.Green Channel"=w432:refnum<vi>)
            n189 = Variant To Data(error in=w437, type=cluster{dbl, dbl} {0.0, 0.0} ("Value"), Variant=w436) -> (data=w430:cluster{dbl, dbl}, error out=w435:errorcluster)
            n190 = property on="Property Node" class="Slide (strict)"(reference=w432, error in=w435, "Value"=w430) -> (error out=w434:errorcluster)  [unwired: 1 out]
          }
          frame "Min.Max.Channel.2" {
            n191 = Variant To Data(error in=w445, type=cluster{dbl, dbl} {0.0, 0.0} ("Value"), Variant=w444) -> (data=w438:cluster{dbl, dbl}, error out=w443:errorcluster)
            n192 = Unbundle By Name(w441) -> ("Equalization.Red Channel"=w440:refnum<vi>)
            n193 = property on="Property Node" class="Slide (strict)"(reference=w440, error in=w443, "Value"=w438) -> (error out=w442:errorcluster)  [unwired: 1 out]
          }
          frame "auto.scale.CH1" {
            n194 = Unbundle By Name(w449) -> ("Equalization.Auto Adjust Green"=w448:refnum<vi>)
            n195 = Variant To Data(error in=w453, type=FALSE ("Value"), Variant=w452) -> (data=w446:bool, error out=w451:errorcluster)
            n196 = property on="Property Node" class="Bool (strict)"(reference=w448, error in=w451, "Value"=w446) -> (error out=w450:errorcluster)  [unwired: 1 out]
          }
          frame "auto.scale.CH.2" {
            n197 = Unbundle By Name(w457) -> ("Equalization.Auto Adjust Red"=w456:refnum<vi>)
            n198 = Variant To Data(error in=w461, type=FALSE ("Value"), Variant=w460) -> (data=w454:bool, error out=w459:errorcluster)
            n199 = property on="Property Node" class="Bool (strict)"(reference=w456, error in=w459, "Value"=w454) -> (error out=w458:errorcluster)  [unwired: 1 out]
          }
          frame "FOCUS" {
            n200 = Unbundle By Name(w462) -> ("Focus Button"=w465:refnum<vi>)
            n201 = Variant To Data(error in=w469, type=FALSE ("Value"), Variant=w468) -> (data=w463:bool, error out=w467:errorcluster)
            n202 = property on="Property Node" class="Bool (strict)"(reference=w465, error in=w467, "Value"=w463) -> (error out=w466:errorcluster)  [unwired: 1 out]
          }
        }
      }
      event Timeout {
        n203 = event-data() -> ()  [unwired: 1 in, 1 out]
      }
    }
    n204 = local read "Exit"() -> (w273:bool)
  }
  n205 = Merge Errors(w4, w5) -> (w2:errorcluster)
  n206 = flat-sequence {
    tunnel: [w473] -> w3
    tunnel: w2 -> [w473]
    tunnel: w1 -> [w471]
    frame #0 {
      n207 = Not(x=w471) -> (.not. x?=w472:bool)
      n208 = local write "Exit"(w472) -> ()
    }
  }
  "error out" <- w3
